vi "gl_Movement correction globals.vi"() -> ()   [LabVIEW 2017]
panel:
  out "Ref size":string
  out "Ref Z-Plane index":i32
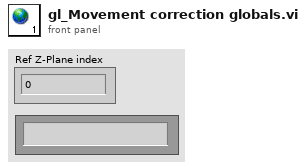
[diagram p1: front panel]
diagram:
